vi "Verify Repository Path.vi"(8 "error in (no error)":errorcluster, 11 "Git in":refnum<class "Git.lvclass">) -> (0 "error out":errorcluster, 3 "Git out":refnum<class "Git.lvclass">)   [LabVIEW 2019, in "Git.lvclass"]
uses:
  Git.lvclass
  Git.lvclass/Git.ctl
  <vilib>/Utility/error.llb/Error Cluster From Error Code.vi
  <vilib>/ErrorRing/Error Ring.xnode
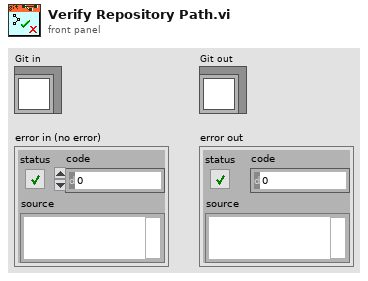
[diagram p1: front panel]
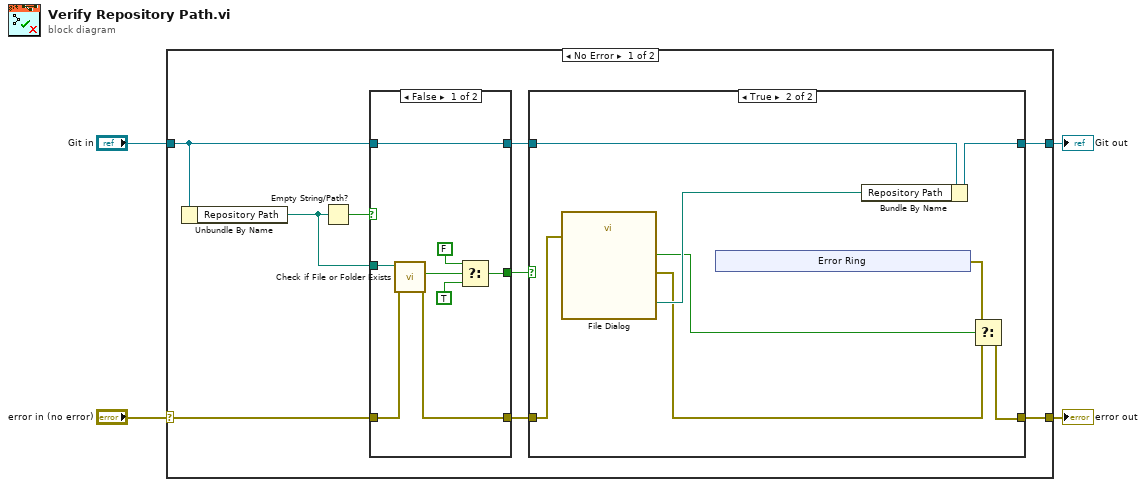
[diagram p0: block diagram]
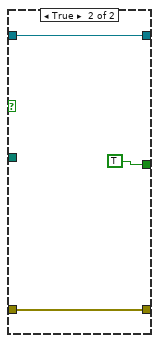
[diagram p2: hidden frame]
diagram:
  n1 = case shown="No Error" "error in (no error)" {
    selector: "error in (no error)" -> [w9 w40]
    tunnel: "Git in" -> [w13 w39]
    tunnel: [w11 w40] -> w3
    tunnel: [w10 w39] -> w2
    frame No Error {
      n2 = Unbundle By Name(w13) -> ("Repository Path"=w12:path)
      n3 = Empty String/Path?(string/path=w12) -> (empty?=w8:bool)
      n4 = case shown="False" w8 {
        tunnel: w13 -> [w18 w24]
        tunnel: w12 -> [w21 _]
        tunnel: [w20 w22] -> w7
        tunnel: w9 -> [w19 w22]
        tunnel: [w18 w24] -> w6
        tunnel: [w16 TRUE] -> w5
        frame False {
          n5 = call <vilib>:"Check if File or Folder Exists.vi"("error in (no error)"=w19, "path"=w21) -> ("error out"=w20:errorcluster, "file or folder exists?"=w17:bool)  [unwired: 7 in, 1 out]
          n6 = Select(t=FALSE, s=w17, f=TRUE) -> (s? t:f=w16:bool)
        }
        frame True {
        }
      }
      n7 = case shown="True" w5 {
        tunnel: w7 -> [w26 w33]
        tunnel: [w26 w27] -> w11
        tunnel: w6 -> [w25 w32]
        tunnel: [w25 w31] -> w10
        frame False {
        }
        frame True {
          n8 = call "File Dialog"("error in"=w33) -> ("selected path"=w34:path, "cancelled"=w28:bool, "error out"=w29:errorcluster)  [unwired: 11 in, 1 out]
          n9 = xnode "Error Ring"() -> ("error out"=w30:errorcluster)
          n10 = Bundle By Name(cluster=w32, "Repository Path"=w34) -> (w31:refnum<class "Git.lvclass">)
          n11 = Select(t=w30, s=w28, f=w29) -> (s? t:f=w27:errorcluster)
        }
      }
    }
    frame Error {
    }
  }
  "Git out" <- w2
  "error out" <- w3
